vi "Establish Comm.vi"(8 "error in (no error)":errorcluster, 11 "VISA resource name":refnum<visa-resource-name>) -> (0 "error out":errorcluster, 3 "VISA resource name out":refnum<visa-resource-name>)   [LabVIEW 2015, in "Spectrometer Digikröm.lvclass"]
uses:
  Digikrom DK24x/Digikrom DK24x.lvlib
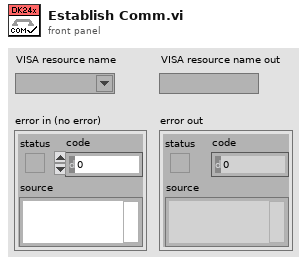
[diagram p1: front panel]
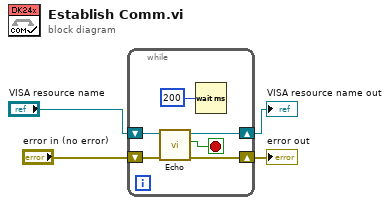
[diagram p0: block diagram]
diagram:
  n1 = while {
    shift-right: [w9] -> w4
    shift-left: "error in (no error)" -> [w8]
    shift-right: [w7] -> w2
    shift-left: "VISA resource name" -> [w6]
    stop <- w5 stop-if-true
    n2 = call "Echo.vi"("error in (no error)"=w8, "VISA resource name"=w6) -> ("error out"=w9:errorcluster, "Comm OK?"=w5:bool, "VISA resource name out"=w7:refnum<visa-resource-name>)  [unwired: 7 in]
    n3 = Wait (ms)(milliseconds to wait=u32 200) -> ()  [unwired: 1 out]
  }
  "VISA resource name out" <- w2
  "error out" <- w4
